vi "Get Attribute STRING.vi"(8 "error in":errorcluster, 10 "Attribute":string, 11 "Config from Excel Table in":refnum<class "Config from Excel Table.lvclass">) -> (0 "error out":errorcluster, 2 "Value":string, 3 "Config from Excel Table out":refnum<class "Config from Excel Table.lvclass">)   [LabVIEW 2025, in "Config from Excel Table.lvclass"]
uses:
  Config from Excel Table.lvclass
  67138228-1a78-4af3-82bc-6e669f4348b6.vi
  67138228-1a78-4af3-82bc-6e669f4348b6.vi/a4169a97-72fc-4003-a778-603cf20cafa0.vi
  <vilib>/JDP Science/JSONtext/Find Item.vi
  <vilib>/JDP Science/JSONtext/Next JSON Value.vi
  <vilib>/JDP Science/JSONtext/String Subset.vi
  <vilib>/JDP Science/JSONtext/Parsing/Advance past next JSON Value (inlined COPY).vi
  <vilib>/JDP Science/JSONtext/Parsing/Advance past whitespace.vi
  <vilib>/JDP Science/JSONtext/Parsing/Advance past String.vi
  <vilib>/JDP Science/JSONtext/Parsing/Advance past Number.vi
  <vilib>/JDP Science/JSONtext/Parsing/Advance past Line Ending.vi
  <vilib>/JDP Science/JSONtext/Is Empty.vi
  <vilib>/JDP Science/JSONtext/Parsing/Parse Full Path or Item Name.vi
  <vilib>/JDP Science/JSONtext/Parsing/Advance past Array.vi
  <vilib>/JDP Science/JSONtext/Parsing/Advance past Object.vi
  <vilib>/JDP Science/JSONtext/support/Error Cluster From Code.vi
  <vilib>/JDP Science/JSONtext/Offset/Find Item Locations by Path.vi
  <vilib>/JDP Science/JSONtext/JSON text to Variant.vi
  Common-LabVIEW-Helpers/Source/errors/-8301 Item not found in JSON--error.vi
  Common-LabVIEW-Helpers/Source/errors/-8300 JSON empty--error.vi
  <vilib>/JDP Science/JSONtext/LVClass Serializer/JSONtext LVClass Serializer.lvclass
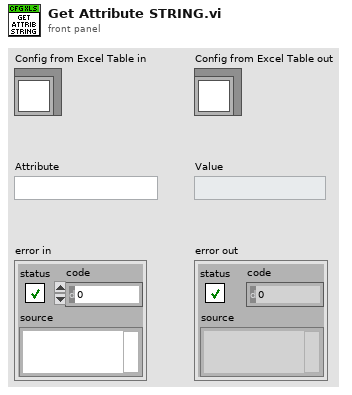
[diagram p1: front panel]
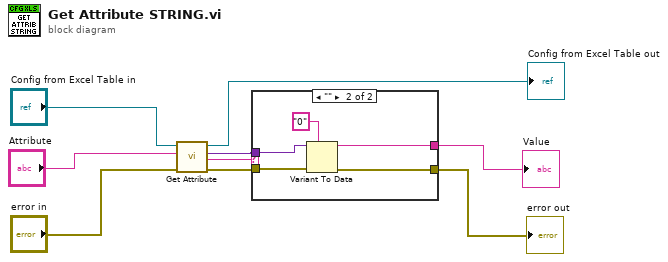
[diagram p0: block diagram]
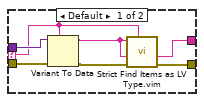
[diagram p2: hidden frame]
diagram:
  n1 = call "Get Attribute.vi"("error in"="error in", "Attribute"="Attribute", "Config from EXCEL Table in"="Config from Excel Table in") -> ("error out"=w5:errorcluster, "Sub Object"=w3:string, "Value"=w4:variant, "Config from EXCEL Table out"=→"Config from Excel Table out":refnum<class "Config from Excel Table.lvclass">)  [unwired: 5 in]
  n2 = case shown="\"\"" w3 {
    selector: w3 -> [w11 _]
    tunnel: [w15 w21] -> w1
    tunnel: [w16 w20] -> w2
    tunnel: w5 -> [w14 w18]
    tunnel: w4 -> [w12 w17]
    frame Default {
      n3 = Variant To Data(error in=w14, type=w11, Variant=w12) -> (data=w10:string, error out=w13:errorcluster)
      n4 = call "Strict Find Items as LV Type.vim"("$Path or Item Name"=w11, "error in"=w13, "Data Type and Default Value"=w10, "<JSON>"=w10) -> ("error out"=w16:errorcluster, "Data out"=w15:string)  [unwired: 5 in, 1 out]
    }
    frame "" {
      n5 = Variant To Data(error in=w18, type="0", Variant=w17) -> (data=w21:string, error out=w20:errorcluster)
    }
  }
  "error out" <- w2
  "Value" <- w1
